vi "Configure_Encoders.vi"(6 "I":dbl, 7 "D":dbl, 9 "P":dbl, 10 "Cluster":T17, 11 "Zero Encoder":bool) -> ()   [LabVIEW 2017]
uses:
  <vilib>/Rock Robotics/WPI/RobotDrive/WPI_RobotDriveDevRef.ctl
  <vilib>/Rock Robotics/WPI/MotorControl/WPI_MotorControlDeviceRef.ctl
  <vilib>/Rock Robotics/WPI/MotorControl/WPI_MotorControlType.ctl
  <vilib>/Rock Robotics/SystemInterfaces/DIO/FPGA_DIOPWMChannel.ctl
  <vilib>/Rock Robotics/WPI/PWM/WPI_PWMDeadband.ctl
  <vilib>/Rock Robotics/SystemInterfaces/DIO/FPGA_DIOChannel.ctl
  TypeDef/CLUSTER_Drive_HW_SRX_Status.ctl
  TypeDef/CLUSTER_4296_SRX_Status.ctl
  TypeDef/CLUSTER_SRX_Status Data.ctl
  TypeDef/CLUSTER_SRX_Encoder Data.ctl
  TypeDef/CLUSTER_SRX_PWM Data.ctl
  TypeDef/CLUSTER_SRX_Analog Data.ctl
  TypeDef/CLUSTER_SRX_Limit Switch Data.ctl
  TypeDef/CLUSTER_SRX_Profile Data.ctl
  TypeDef/ENUM_Drive_ACT Loop_Mode.ctl
  TypeDef/CLUSTER_Left and Right.ctl
  Public/Documents/Cross The Road Electronics/Phoenix-LabVIEW/Motor Controller/Get/CTRE_Phoenix_MotorController_GetSelectedSensorData.vi
  Global_WC_Drive_Encoder_Values.vi
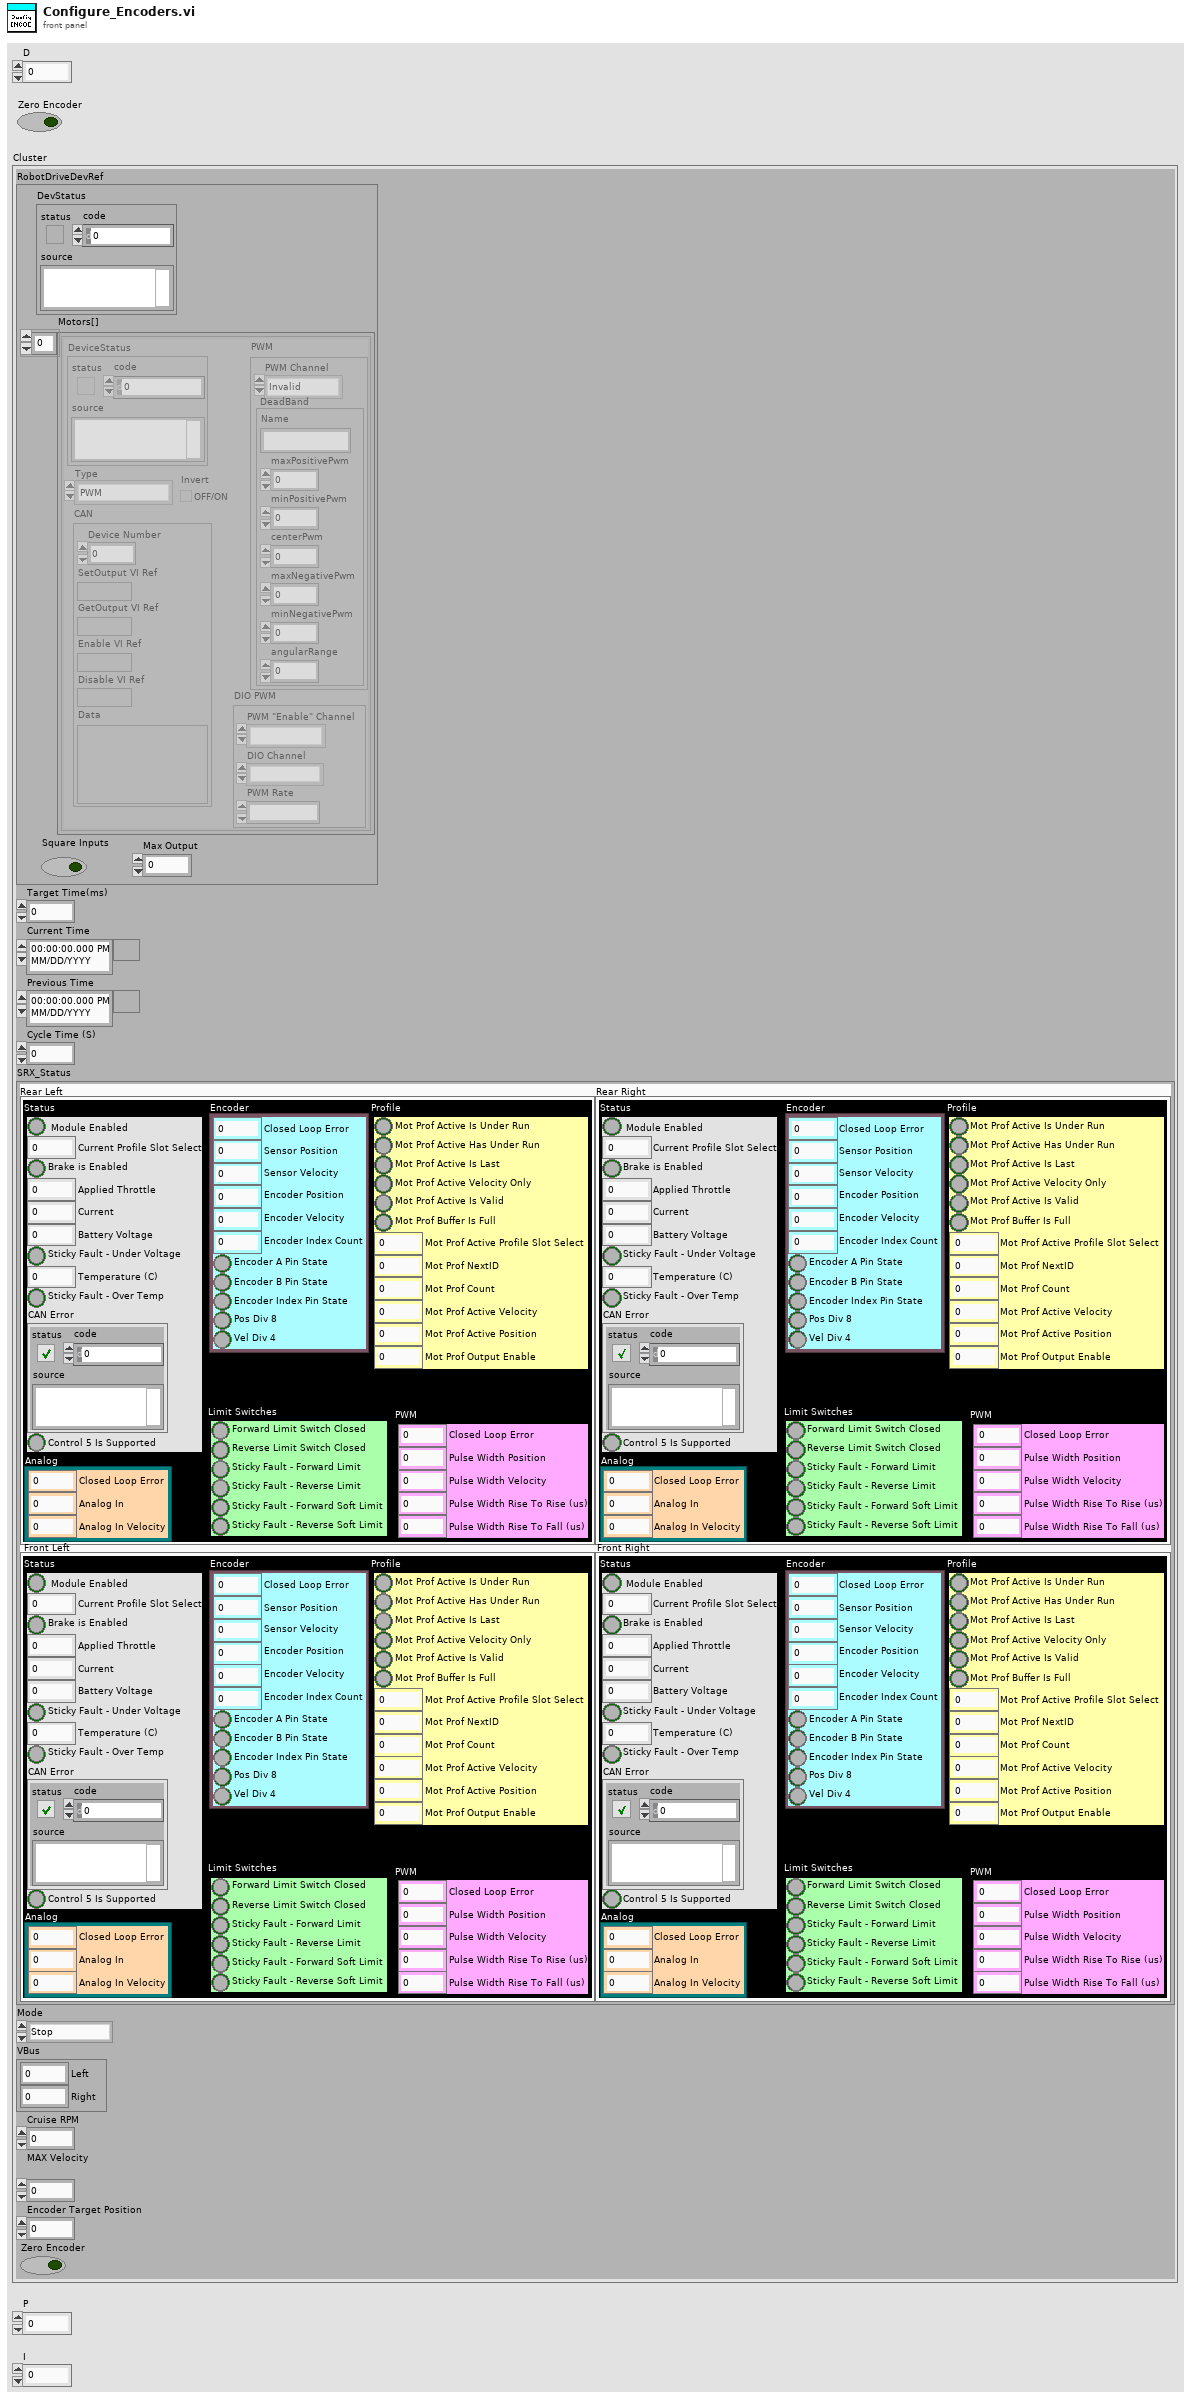
[diagram p1: front panel]
types:
  T1 = typedef "WPI_RobotDriveDevRef.ctl" = cluster{"DevStatus":errorcluster, "Motors[]":T2[], "Square Inputs":bool, "Max Output":dbl}
  T2 = typedef "WPI_MotorControlDeviceRef.ctl" = cluster{"DeviceStatus":errorcluster, "Type":T3, "PWM":cluster{"PWM Channel":T4, "DeadBand":T5}, "CAN":cluster{"Device Number":u8, "SetOutput VI Ref":variant, "GetOutput VI Ref":variant, "Enable VI Ref":variant, "Disable VI Ref":variant, "Data":variant}, "Invert":bool, "DIO PWM":cluster{"PWM \"Enable\" Channel":T4, "DIOChannel":T6, "PWM Rate":dbl}}
  T3 = typedef "WPI_MotorControlType.ctl" = enum16{"PWM", "CAN", "DIO PWM"}
  T4 = typedef "FPGA_DIOPWMChannel.ctl" = enum8{"PWM 0", "PWM 1", "PWM 2", "PWM 3", "PWM 4", "PWM 5", "PWM 6", "PWM 7", "PWM 8", "PWM 9", "PWM MXP 0", "PWM MXP 1", "PWM MXP 2", "PWM MXP 3", "PWM MXP 4", "PWM MXP 5", "PWM MXP 6", "PWM MXP 7", "PWM MXP 8", "PWM MXP 9", "Invalid"}
  T5 = typedef "WPI_PWMDeadband.ctl" = cluster{"Name":string, "maxPositivePwm":i32, "minPositivePwm":i32, "centerPwm":i32, "maxNegativePwm":i32, "minNegativePwm":i32, "angularRange":u16}
  T6 = typedef "FPGA_DIOChannel.ctl" = enum8{"DIO 0", "DIO 1", "DIO 2", "DIO 3", "DIO 4", "DIO 5", "DIO 6", "DIO 7", "DIO 8", "DIO 9", "DIO MXP 0", "DIO MXP 1", "DIO MXP 2", "DIO MXP 3", "DIO MXP 4", "DIO MXP 5", "DIO MXP 6", "DIO MXP 7", "DIO MXP 8", "DIO MXP 9", "DIO MXP 10", "DIO MXP 11", "DIO MXP 12", "DIO MXP 13", "DIO MXP 14", "DIO MXP 15", "SPI Port CS1", "SPI Port CS2", "SPI Port CS3", "SPI Port MISO", "SPI Port MOSI", "Invalid"}
  T7 = typedef "CLUSTER_Drive_HW_SRX_Status.ctl" = cluster{"Rear Left":T8, "Rear Right":T8, "Front Left":T8, "Front Right":T8}
  T8 = typedef "CLUSTER_4296_SRX_Status.ctl" = cluster{"Status":T9, "Encoder":T10, "PWM ":T11, "Analog":T12, "Limit Switches":T13, "Profile":T14}
  T9 = typedef "CLUSTER_SRX_Status Data.ctl" = cluster{"Module Enabled":bool, "Current Profile Slot Select":dbl, "Brake is Enabled":bool, "Applied Throttle":dbl, "Current":dbl, "Battery Voltage":dbl, "Sticky Fault - Under Voltage":bool, "Temperature (C)":dbl, "Sticky Fault - Over Temp":bool, "CAN Error":errorcluster, "Control 5 Is Supported":bool}
  T10 = typedef "CLUSTER_SRX_Encoder Data.ctl" = cluster{"Closed Loop Error":dbl, "Sensor Position":dbl, "Sensor Velocity":dbl, "Encoder Position":dbl, "Encoder Velocity":dbl, "Encoder Index Count":dbl, "Encoder A Pin State":bool, "Encoder B Pin State":bool, "Encoder Index Pin State":bool, "Pos Div 8":bool, "Vel Div 4":bool}
  T11 = typedef "CLUSTER_SRX_PWM Data.ctl" = cluster{"Closed Loop Error":dbl, "Pulse Width Position":i32, "Pulse Width Velocity":i32, "Pulse Width Rise To Rise (us)":i32, "Pulse Width Rise To Fall (us)":i32}
  T12 = typedef "CLUSTER_SRX_Analog Data.ctl" = cluster{"Closed Loop Error":dbl, "Analog In":dbl, "Analog In Velocity":dbl}
  T13 = typedef "CLUSTER_SRX_Limit Switch Data.ctl" = cluster{"Forward Limit Switch Closed":bool, "Reverse Limit Switch Closed":bool, "Sticky Fault - Forward Limit":bool, "Sticky Fault - Reverse Limit":bool, "Sticky Fault - Forward Soft Limit":bool, "Sticky Fault - Reverse Soft Limit":bool}
  T14 = typedef "CLUSTER_SRX_Profile Data.ctl" = cluster{"Mot Prof Active Is Under Run":bool, "Mot Prof Active Has Under Run":bool, "Mot Prof Active Is Last":bool, "Mot Prof Active Velocity Only":bool, "Mot Prof Active Is Valid":bool, "Mot Prof Buffer Is Full":bool, "Mot Prof Active Profile Slot Select":i32, "Mot Prof NextID":i32, "Mot Prof Count":i32, "Mot Prof Active Velocity":dbl, "Mot Prof Active Position":dbl, "Mot Prof Output Enable":i32}
  T15 = typedef "ENUM_Drive_ACT Loop_Mode.ctl" = enum16{"Stop", "Position", "VBus", "Profile"}
  T16 = typedef "CLUSTER_Left and Right.ctl" = cluster{"Left":dbl, "Right":dbl}
  T17 = cluster{"RobotDriveDevRef":T1, "Target Time(ms)":u32, "Current Time":timestamp, "Previous Time":timestamp, "Cycle Time (S)":dbl, "SRX_Status":T7, "Mode":T15, "VBus":T16, "Cruise RPM":dbl, "MAX Velocity\n":dbl, "Encoder Target Position":i32, "Zero Encoder":bool}
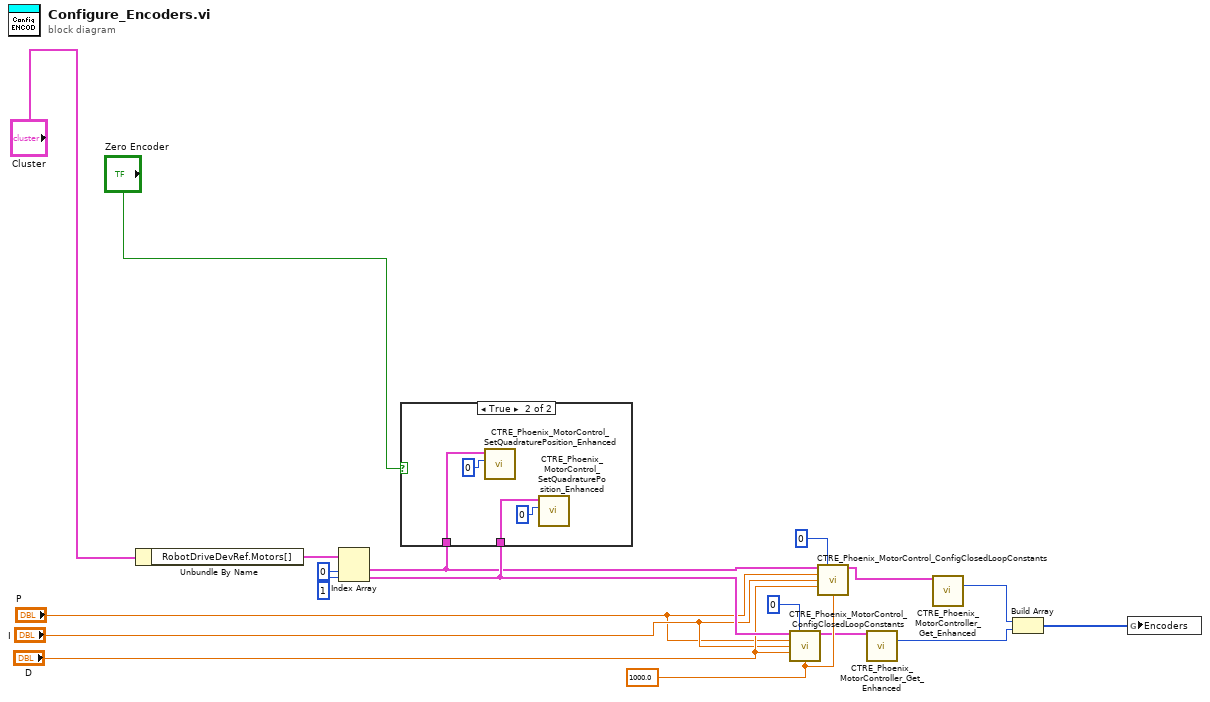
[diagram p0: block diagram]
diagram:
  w18 = 1000.0
  n1 = Unbundle By Name("Cluster") -> ("RobotDriveDevRef.Motors[]"=w1:T2[])
  n2 = Index Array(array=w1, index #1=0 ("index"), index #2=1 ("index")) -> (element #1=w15:T2, element #2=w16:T2)
  n3 = case shown="True" "Zero Encoder" {
    tunnel: w15 -> [_ w22]
    tunnel: w16 -> [_ w19]
    frame False {
    }
    frame True {
      n4 = call "CTRE_Phoenix_MotorControl_SetQuadraturePosition_Enhanced.vi"("New Position"=0, "PhoenixMotorControlDevRef"=w22) -> ()  [unwired: 8 in, 2 out]
      n5 = call "CTRE_Phoenix_MotorControl_SetQuadraturePosition_Enhanced.vi"("New Position"=0, "PhoenixMotorControlDevRef"=w19) -> ()  [unwired: 8 in, 2 out]
    }
  }
  n6 = call "CTRE_Phoenix_MotorControl_ConfigClosedLoopConstants.vi"("PhoenixMotorControlDevRef"=w16, "slotIdx"=0, "P"="P", "I"="I", "D"="D", "I Zone"=w18) -> ("PhoenixMotorControlDevRef"=w11:T2)  [unwired: 8 in, 1 out]
  n7 = call "CTRE_Phoenix_MotorControl_ConfigClosedLoopConstants.vi"("PhoenixMotorControlDevRef"=w15, "slotIdx"=0, "P"="P", "I"="I", "D"="D", "I Zone"=w18) -> ("PhoenixMotorControlDevRef"=w10:T2)  [unwired: 8 in, 1 out]
  n8 = call-poly "CTRE_Phoenix_MotorController_Get_Enhanced.vi"("PhoenixMotorControlDevRef"=w11) -> ("Position (Raw Sensor Units)"=w6:i32)  [unwired: 11 in, 3 out]
  n9 = call-poly "CTRE_Phoenix_MotorController_Get_Enhanced.vi"("PhoenixMotorControlDevRef"=w10) -> ("Position (Raw Sensor Units)"=w5:i32)  [unwired: 11 in, 3 out]
  n10 = Build Array(w5, w6) -> (w7:i32[])
  n11 = global write "Global_WC_Drive_Encoder_Values.vi" "Encoders"(w7) -> ()
